vi "Read Power Supply.vi"(7 "1-Wire DIO Pin":refnum<k21>, 8 "error in (no error)":errorcluster) -> (0 "error out":errorcluster, 2 "All Devices Powered?":bool)   [LabVIEW 2014, in "Maxim 1-Wire.lvlib"]
doc: "READ POWER SUPPLY [B4h]\nThe master device issues this command followed by a read time slot to determine if any DS18B20s on the bus are using parasite power. During the read time slot, parasite powered DS18B20s will pull the bus low, and externally powered DS18B20s will let the bus remain high."
uses:
  Maxim 1-Wire.lvlib
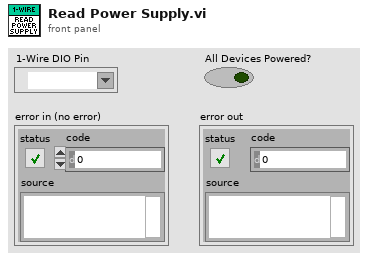
[diagram p1: front panel]
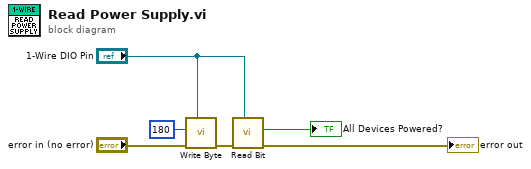
[diagram p0: block diagram]
diagram:
  n1 = call "Write Byte.vi"("1-Wire DIO Pin"="1-Wire DIO Pin", "error in"="error in (no error)", "Tx data"=u8 180 ("Tx data 2")) -> ("error out"=w3:errorcluster)  [unwired: 8 in]
  n2 = call "Read Bit.vi"("1-Wire DIO Pin"="1-Wire DIO Pin", "error in"=w3) -> ("error out"=→"error out":errorcluster, "Bit Read"=→"All Devices Powered?":bool)  [unwired: 8 in]
